vi "AlliGator Get n-Exp Guess Parameters.vi"(8 "Error In":errorcluster, 9 "IRF":cluster{"t Array":dbl[], "Y Array":dbl[]}, 10 "Decay":cluster{"t Array":dbl[], "Y Array":dbl[]}, 11 "Fit Model":T1 caption="Model") -> (0 "Error Out":errorcluster, 1 "Guess Parameters Options":T2, 3 "Guess Parameters":dbl[](array[numeric]))   [LabVIEW 2021, in "AlliGator Decay Fit.lvlib"]
doc: "Get numerically estimated <B>Guess Parameters</B> for 1-Exp or 2-Exp models."
uses:
  AlliGator Decay Fit.lvlib
  AlliGator Guess Parameters Options.ctl
  Fits/Decay Convolution/Decay Model.ctl
  Fits/Fits.lvlib
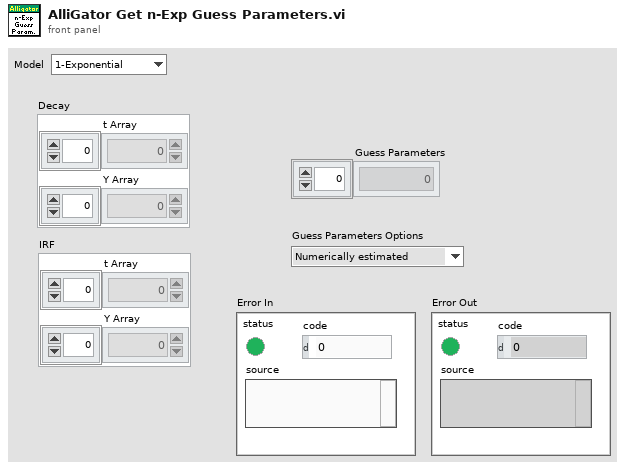
[diagram p1: front panel]
types:
  T1 = typedef "Fits.lvlib/Decay Model.ctl" = enum16{"1-Exponential", "2-Exponentials"}
  T2 = typedef "AlliGator Decay Fit.lvlib/AlliGator Guess Parameters Options.ctl" = enum16{"Numerically estimated", "User-provided", "User-provided (normalized)", "Last valid fitted parameters"}
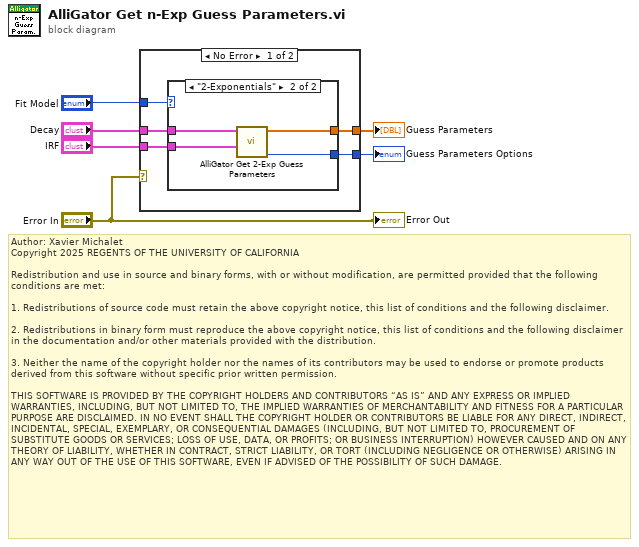
[diagram p0: block diagram]
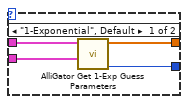
[diagram p2: hidden frame]
diagram:
  # "Author: Xavier Michalet\nCopyright 2025 REGENTS OF THE UNIVERSITY OF CALIFORNIA\n\nRedistribution and use in source and binary forms, with or without modification, are permitted provided that the following conditions are met:\n\n1. Redistributions of source code must retain the above copyright notice, this list of conditions and the following disclaimer.\n\n2. Redistributions in binary form must reproduce the above copyright notice, this list of conditions and the following disclaimer in the documentation and/or other materials provided with the distribution.\n\n3. Neither the name of the copyright holder nor the names of its contributors may be used to endorse or promote products derived from this software without specific prior written permission.\n\nTHIS SOFTWARE IS PROVIDED BY THE COPYRIGHT HOLDERS AND CONTRIBUTORS “AS IS” AND ANY EXPRESS OR IMPLIED WARRANTIES, INCLUDING, BUT NOT LIMITED TO, THE IMPLIED WARRANTIES OF MERCHANTABILITY AND FITNESS FOR A PARTICULAR PURPOSE ARE DISCLAIMED. IN NO EVENT SHALL THE COPYRIGHT HOLDER OR CONTRIBUTORS BE LIABLE FOR ANY DIRECT, INDIRECT, INCIDENTAL, SPECIAL, EXEMPLARY, OR CONSEQUENTIAL DAMAGES (INCLUDING, BUT NOT LIMITED TO, PROCUREMENT OF SUBSTITUTE GOODS OR SERVICES; LOSS OF USE, DATA, OR PROFITS; OR BUSINESS INTERRUPTION) HOWEVER CAUSED AND ON ANY THEORY OF LIABILITY, WHETHER IN CONTRACT, STRICT LIABILITY, OR TORT (INCLUDING NEGLIGENCE OR OTHERWISE) ARISING IN ANY WAY OUT OF THE USE OF THIS SOFTWARE, EVEN IF ADVISED OF THE POSSIBILITY OF SUCH DAMAGE."
  n1 = case shown="No Error" "Error In" {
    tunnel: [w11 _] -> w6
    tunnel: "IRF" -> [w10 _]
    tunnel: "Decay" -> [w9 _]
    tunnel: "Fit Model" -> [w8 _]
    tunnel: [w7 _] -> w2
    frame No Error {
      n2 = case shown="\"2-Exponentials\"" w8 {
        tunnel: [w12 w16] -> w7
        tunnel: [w15 w19] -> w11
        tunnel: w10 -> [w14 w18]
        tunnel: w9 -> [w13 w17]
        frame "1-Exponential", Default {
          n3 = call "AlliGator Get 1-Exp Guess Parameters.vi"("IRF"=w14, "Decay"=w13) -> ("Guess Parameters Type"=w12:T2, "Guess Parameters"=w15:dbl[])  [unwired: 7 in, 1 out]
        }
        frame "2-Exponentials" {
          n4 = call "AlliGator Get 2-Exp Guess Parameters.vi"("IRF"=w18, "Decay"=w17) -> ("Guess Parameters Type"=w16:T2, "Guess Parameters"=w19:dbl[])  [unwired: 7 in, 1 out]
        }
      }
    }
    frame Error {
    }
  }
  "Guess Parameters Options" <- w2
  "Guess Parameters" <- w6
  "Error Out" <- "Error In"
